vi "Log VI.vi"(11 "DVR":T1) -> ()   [LabVIEW 2015, in "System Log.lvclass"]
uses:
  System Log.lvclass
  Controls/DVR.ctl
  System Log.lvclass/System Log.ctl
  Accessors/Read sysLogQueue.vi
panel:
  in  "clear":bool
  out "sysLog":string[][](table)
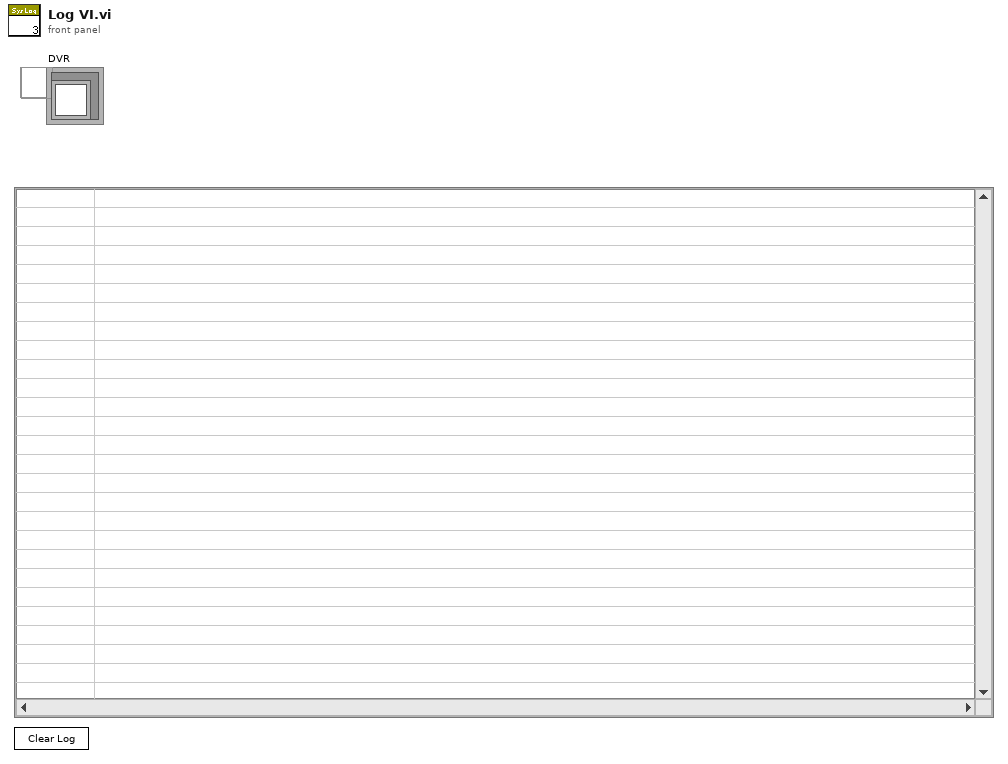
[diagram p1: front panel]
types:
  T1 = typedef "System Log.lvclass/DVR.ctl" = refnum<data-value>
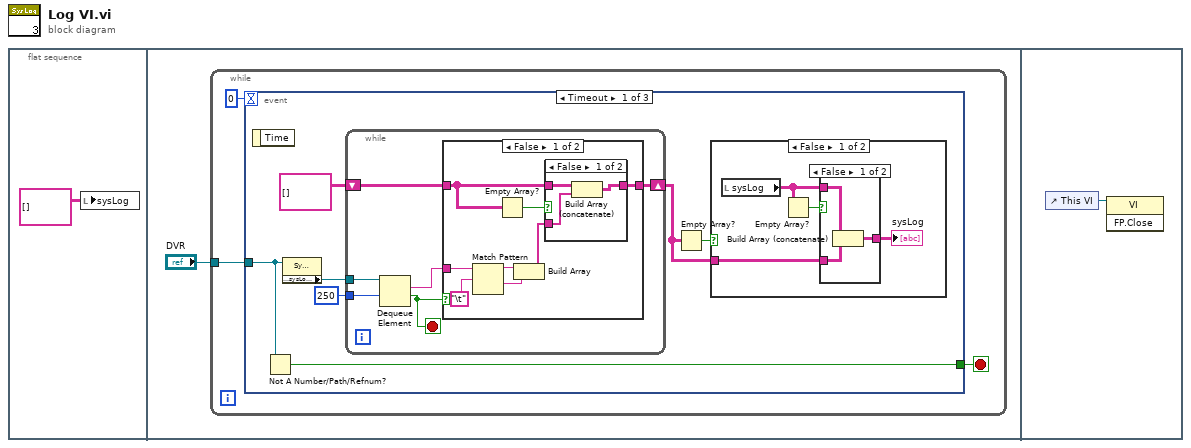
[diagram p0: block diagram]
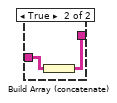
[diagram p2: hidden frame]
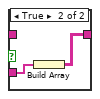
[diagram p4: hidden frame]
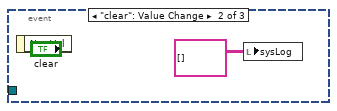
[diagram p6: hidden frame]
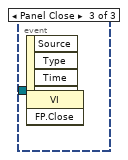
[diagram p7: hidden frame]
diagram:
  n1 = flat-sequence {
    frame #0 {
      n2 = local write "sysLog"(string[][] [] ("sysLog")) -> ()
    }
    frame #1 {
      n3 = while {
        tunnel: "DVR" -> [w5]
        stop <- w3 stop-if-true
        n4 = event shown="[0] Timeout" {
          selector: _ -> [_ _ _]
          dyn-events: _ -> [_ _ _]
          timeout: 0 -> [_ _ _]
          tunnel: w5 -> [w9 _ _]
          tunnel: [w8 _ _] -> w3
          event Timeout {
            n5 = event-data() -> ()  [unwired: 1 in, 1 out]
            n6 = Not A Number/Path/Refnum?(number/path/refnum=w9) -> (NaN/Path/Refnum?=w8:bool)
            n7 = property class="Sys Log"(reference=w9) -> ("Accessors:sysLogQueue"=w12:refnum<queue>)  [unwired: 1 in, 2 out]
            n8 = while {
              tunnel: w12 -> [w27]
              tunnel: 250 ("timeout in ms (-1)") -> [w26]
              shift-right: [w22] -> w6
              shift-left: string[][] [] -> [w23]
              stop <- w24 stop-if-true
              n9 = Dequeue Element(queue=w27, timeout in ms (-1)=w26) -> (element=w25:string, timed out?=w24:bool)  [unwired: 1 in, 2 out]
              n10 = case shown="False" w24 {
                tunnel: w25 -> [w35 _]
                tunnel: w23 -> [w28 w41]
                tunnel: [w29 w41] -> w22
                frame False {
                  n11 = Match Pattern(string=w35, regular expression="\t") -> (before substring=w33:string, after substring=w32:string)  [unwired: 1 in, 2 out]
                  n12 = Empty Array?(array=w28) -> (empty?=w31:bool)
                  n13 = Build Array(w33, w32) -> (w30:string[])
                  n14 = case shown="False" w31 {
                    tunnel: w30 -> [w37 w40]
                    tunnel: [w36 w39] -> w29
                    tunnel: w28 -> [w38 _]
                    frame False {
                      n15 = Build Array (concatenate)(w38, w37) -> (w36:string[][])
                    }
                    frame True {
                      n16 = Build Array(w40) -> (w39:string[][])
                    }
                  }
                }
                frame True {
                }
              }
            }
            n17 = Empty Array?(array=w6) -> (empty?=w10:bool)
            n18 = case shown="False" w10 {
              tunnel: w6 -> [w15 _]
              frame False {
                n19 = local read "sysLog"() -> (w13:string[][])
                n20 = Empty Array?(array=w13) -> (empty?=w16:bool)
                n21 = case shown="False" w16 {
                  tunnel: w15 -> [w18 w21]
                  tunnel: [w17 w20] -> w14
                  tunnel: w13 -> [w19 _]
                  frame False {
                    n22 = Build Array (concatenate)(w19, w18) -> (w17:string[][])
                  }
                  frame True {
                    n23 = Build Array (concatenate)(w21) -> (w20:string[][])
                  }
                }
                "sysLog" <- w14
              }
              frame True {
              }
            }
          }
          event "clear": Value Change {
            n24 = event-data() -> ()  [unwired: 1 in, 1 out]
            n25 = local write "sysLog"(string[][] [] ("sysLog")) -> ()
          }
          event Panel Close {
            n26 = event-data() -> ("VIRef"=w43:refnum<vi>)  [unwired: 1 in, 3 out]
            n27 = invoke class="VI" method="FP.Close"(reference=w43) -> ()  [unwired: 2 in, 3 out]
          }
        }
      }
    }
    frame #2 {
      n28 = control-ref of="This VI"() -> (w44:refnum<vi>)
      n29 = invoke class="VI" method="FP.Close"(reference=w44) -> ()  [unwired: 2 in, 3 out]
    }
  }
